vi "Main.vi"() -> ()   [LabVIEW 2019, in "OCVTest.lvlib" / "OCVTest.lvclass"]
uses:
  OCVTest.lvclass
  typeDefs/Server State Data.ctl
  OCVTest.lvclass/OCVTest.ctl
panel:
  in  "Stop":bool
  in  "Enable Async Mode":bool
  in  "Server Address":string="0.0.0.0.50051"
  in  "Server Certificate File (.crt)":path
  in  "Server Key File (.key)":path
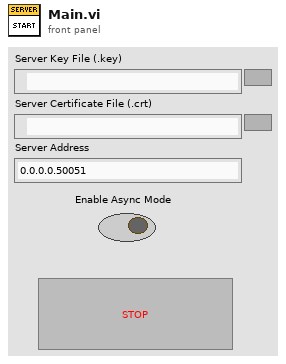
[diagram p1: front panel]
types:
  T1 = typedef "OCVTest.lvlib/OCVTest.lvclass/Server State Data.ctl" = cluster{"Data":string}
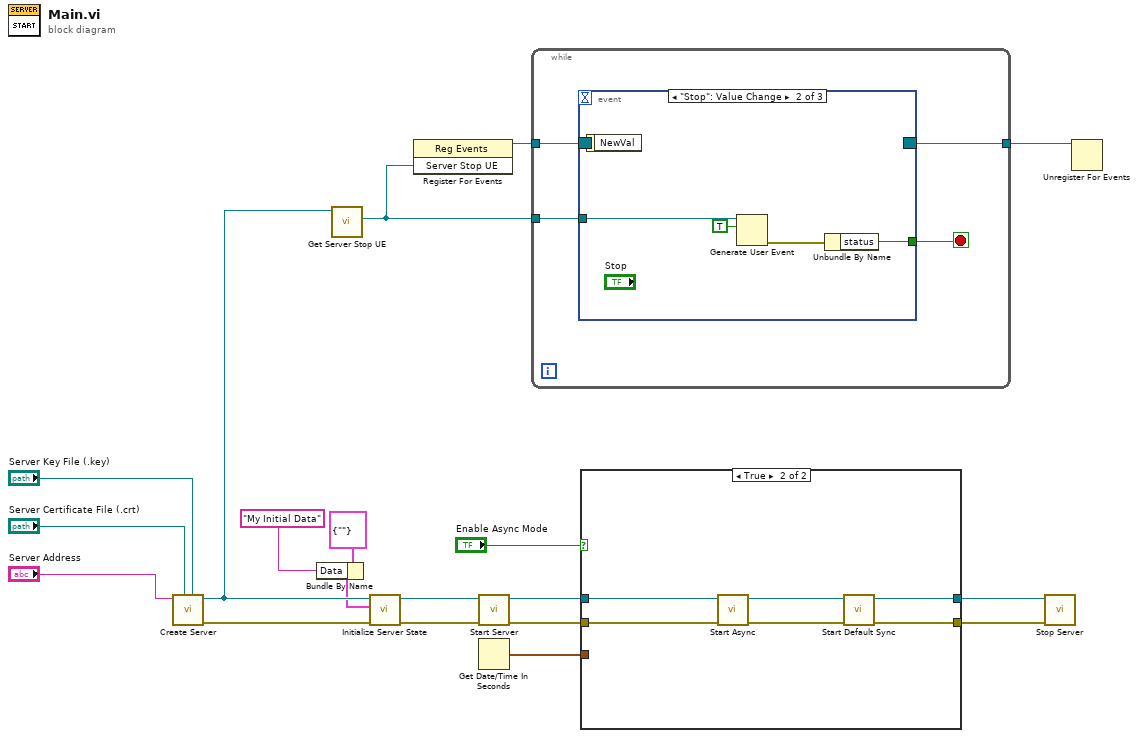
[diagram p0: block diagram]
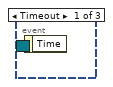
[diagram p2: hidden frame]
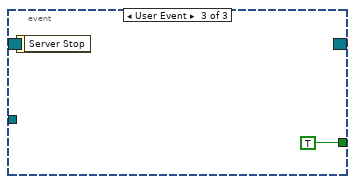
[diagram p3: hidden frame]
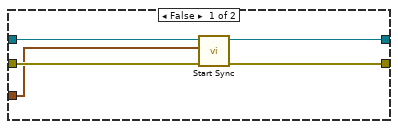
[diagram p4: hidden frame]
diagram:
  n1 = call "Create Server.vi"("Server Key File (.key)"="Server Key File (.key)", "Server Certificate File (.crt)"="Server Certificate File (.crt)", "Server Address"="Server Address") -> ("error out"=w8:errorcluster, "gRPC Server out"=w5:refnum<class "OCVTest.lvclass">)  [unwired: 7 in]
  n2 = Bundle By Name(cluster=T1 {"Data"=""} ("Initial State"), "Data"="My Initial Data") -> (w3:T1)
  n3 = call "Get Server Stop UE.vi"("OOP Server in"=w5) -> ("Server Stop UE"=w9:refnum<user-event>)  [unwired: 9 in, 1 out]
  n4 = call "Initialize Server State.vi"("error in (no error)"=w8, "Initial State"=w3, "gRPC Server in"=w5) -> ("error out"=w7:errorcluster, "gRPC Server out"=w6:refnum<class "OCVTest.lvclass">)  [unwired: 7 in]
  n5 = register-events(w9) -> (reference out=w11:refnum<event-registration>)  [unwired: 2 in, 1 out]
  n6 = call "Start Server.vi"("error in (no error)"=w7, "gRPC Server in"=w6) -> ("error out"=w19:errorcluster, "gRPC Server out"=w18:refnum<class "OCVTest.lvclass">)  [unwired: 8 in]
  n7 = Get Date/Time In Seconds() -> (seconds since 1Jan1904=w1:timestamp)
  n8 = while {
    tunnel: w9 -> [w23]
    tunnel: w11 -> [w22]
    tunnel: [w20] -> w10
    stop <- w21 stop-if-true
    n9 = event shown="[1] \"Stop\": Value Change" {
      selector: w22 -> [_ _ _]
      dyn-events: [_ _ _] -> w20
      timeout: _ -> [_ _ _]
      tunnel: w23 -> [_ w27 _]
      tunnel: [_ w24 TRUE] -> w21
      event Timeout {
        n10 = event-data() -> ()  [unwired: 1 in, 1 out]
      }
      event "Stop": Value Change {
        n11 = event-data() -> ()  [unwired: 1 in, 1 out]
        n12 = Generate User Event(user event=w27, event data cluster=TRUE ("event data")) -> (error out=w25:errorcluster)  [unwired: 2 in, 1 out]
        n13 = Unbundle By Name(w25) -> ("status"=w24:bool)
      }
      event User Event {
        n14 = event-data() -> ()  [unwired: 1 in, 1 out]
      }
    }
  }
  n15 = case shown="True" "Enable Async Mode" {
    tunnel: w19 -> [w33 w39]
    tunnel: w18 -> [w32 w38]
    tunnel: [w31 w35] -> w17
    tunnel: [w30 w34] -> w16
    tunnel: w1 -> [w29 _]
    frame False {
      n16 = call "Start Sync.vi"("error in (no error)"=w33, "current time"=w29, "gRPC Server in"=w32) -> ("error out"=w31:errorcluster, "gRPC Server out"=w30:refnum<class "OCVTest.lvclass">)  [unwired: 7 in]
    }
    frame True {
      n17 = call "Start Async.vi"("error in (no error)"=w39, "gRPC Server in"=w38) -> ("error out"=w36:errorcluster, "gRPC Server out"=w37:refnum<class "OCVTest.lvclass">)  [unwired: 8 in]
      n18 = call "Start Default Sync.vi"("error in (no error)"=w36, "gRPC Server in"=w37) -> ("error out"=w35:errorcluster, "gRPC Server out"=w34:refnum<class "OCVTest.lvclass">)  [unwired: 8 in]
    }
  }
  n19 = call "Stop Server.vi"("error in (no error)"=w17, "gRPC Server in"=w16) -> ()  [unwired: 9 in, 1 out]
  n20 = Unregister For Events(event registration refnum=w10) -> ()  [unwired: 1 in, 1 out]
